vi "saveBuildHeader_poly.vi"   [LabVIEW 2011]
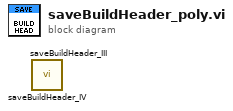
[diagram p0: block diagram]
diagram:
  n1 = call "saveBuildHeader_IV.vi"() -> ()  [unwired: 10 in, 2 out]
  n2 = call "saveBuildHeader_III.vi"() -> ()  [unwired: 10 in, 2 out]
